vi "Buzzer.vi"   [LabVIEW 2022 SP3]
uses:
  <vilib>/DAQmx/write.llb/DAQmx Write (Digital Bool 1Line 1Point).vi
  <vilib>/DAQmx/create/channels.llb/DAQmx Create Channel (DO-Digital Output).vi
  <vilib>/DAQmx/miscellaneous.llb/DAQmx Fill In Error Info.vi
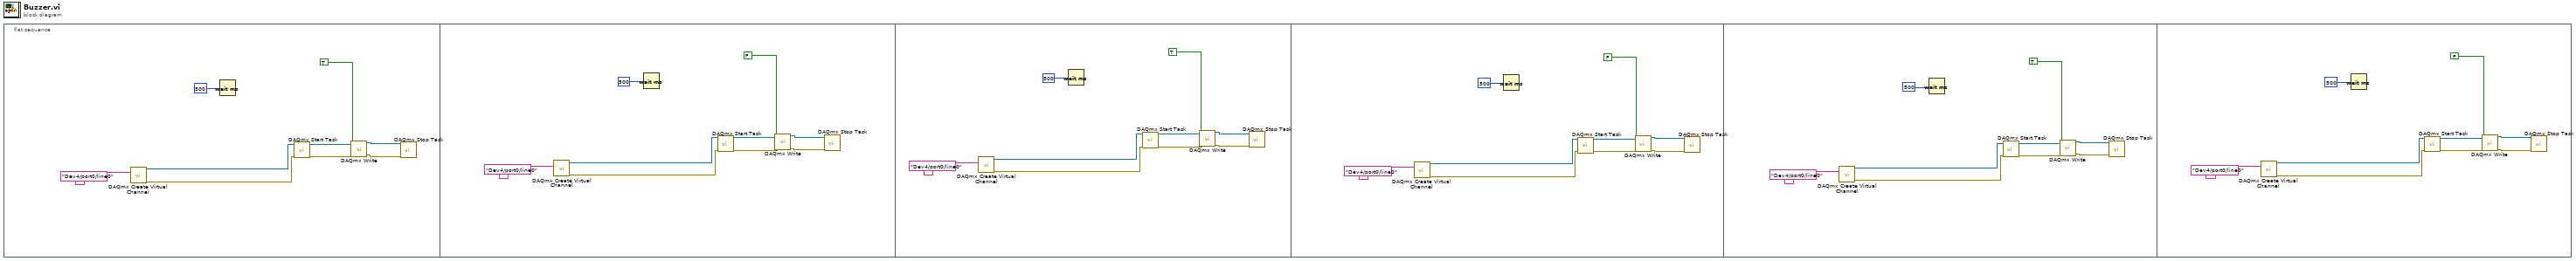
[diagram p0: block diagram]
diagram:
  n1 = flat-sequence {
    frame #0 {
      n2 = call-poly <vilib>:"DAQmx Create Virtual Channel.vi"("lines"=tag "Dev4/port0/line0" ("DAQmx Physical Channel")) -> ("task out"=w1:refnum<k21>, "error out"=w2:errorcluster)  [unwired: 13 in]
      n3 = Wait (ms)(milliseconds to wait=u32 500 ("millisecond timer value")) -> ()  [unwired: 1 out]
      n4 = call <vilib>:"DAQmx Start Task.vi"("task/channels in"=w1, "error in"=w2) -> ("task out"=w8:refnum<k21>, "error out"=w7:errorcluster)  [unwired: 12 in]
      n5 = call-poly <vilib>:"DAQmx Write.vi"("task/channels in"=w8, "data"=TRUE, "error in"=w7) -> ("task out"=w5:refnum<k21>, "error out"=w4:errorcluster)  [unwired: 10 in, 1 out]
      n6 = call <vilib>:"DAQmx Stop Task.vi"("task/channels in"=w5, "error in"=w4) -> ()  [unwired: 12 in, 2 out]
    }
    frame #1 {
      n7 = call-poly <vilib>:"DAQmx Create Virtual Channel.vi"("lines"=tag "Dev4/port0/line0" ("DAQmx Physical Channel")) -> ("task out"=w10:refnum<k21>, "error out"=w11:errorcluster)  [unwired: 13 in]
      n8 = Wait (ms)(milliseconds to wait=u32 500 ("millisecond timer value")) -> ()  [unwired: 1 out]
      n9 = call <vilib>:"DAQmx Start Task.vi"("task/channels in"=w10, "error in"=w11) -> ("task out"=w17:refnum<k21>, "error out"=w16:errorcluster)  [unwired: 12 in]
      n10 = call-poly <vilib>:"DAQmx Write.vi"("task/channels in"=w17, "data"=FALSE, "error in"=w16) -> ("task out"=w14:refnum<k21>, "error out"=w13:errorcluster)  [unwired: 10 in, 1 out]
      n11 = call <vilib>:"DAQmx Stop Task.vi"("task/channels in"=w14, "error in"=w13) -> ()  [unwired: 12 in, 2 out]
    }
    frame #2 {
      n12 = call-poly <vilib>:"DAQmx Create Virtual Channel.vi"("lines"=tag "Dev4/port0/line0" ("DAQmx Physical Channel")) -> ("task out"=w19:refnum<k21>, "error out"=w20:errorcluster)  [unwired: 13 in]
      n13 = Wait (ms)(milliseconds to wait=u32 500 ("millisecond timer value")) -> ()  [unwired: 1 out]
      n14 = call <vilib>:"DAQmx Start Task.vi"("task/channels in"=w19, "error in"=w20) -> ("task out"=w26:refnum<k21>, "error out"=w25:errorcluster)  [unwired: 12 in]
      n15 = call-poly <vilib>:"DAQmx Write.vi"("task/channels in"=w26, "data"=TRUE, "error in"=w25) -> ("task out"=w23:refnum<k21>, "error out"=w22:errorcluster)  [unwired: 10 in, 1 out]
      n16 = call <vilib>:"DAQmx Stop Task.vi"("task/channels in"=w23, "error in"=w22) -> ()  [unwired: 12 in, 2 out]
    }
    frame #3 {
      n17 = call-poly <vilib>:"DAQmx Create Virtual Channel.vi"("lines"=tag "Dev4/port0/line0" ("DAQmx Physical Channel")) -> ("task out"=w28:refnum<k21>, "error out"=w29:errorcluster)  [unwired: 13 in]
      n18 = Wait (ms)(milliseconds to wait=u32 500 ("millisecond timer value")) -> ()  [unwired: 1 out]
      n19 = call <vilib>:"DAQmx Start Task.vi"("task/channels in"=w28, "error in"=w29) -> ("task out"=w35:refnum<k21>, "error out"=w34:errorcluster)  [unwired: 12 in]
      n20 = call-poly <vilib>:"DAQmx Write.vi"("task/channels in"=w35, "data"=FALSE, "error in"=w34) -> ("task out"=w32:refnum<k21>, "error out"=w31:errorcluster)  [unwired: 10 in, 1 out]
      n21 = call <vilib>:"DAQmx Stop Task.vi"("task/channels in"=w32, "error in"=w31) -> ()  [unwired: 12 in, 2 out]
    }
    frame #4 {
      n22 = call-poly <vilib>:"DAQmx Create Virtual Channel.vi"("lines"=tag "Dev4/port0/line0" ("DAQmx Physical Channel")) -> ("task out"=w37:refnum<k21>, "error out"=w38:errorcluster)  [unwired: 13 in]
      n23 = Wait (ms)(milliseconds to wait=u32 500 ("millisecond timer value")) -> ()  [unwired: 1 out]
      n24 = call <vilib>:"DAQmx Start Task.vi"("task/channels in"=w37, "error in"=w38) -> ("task out"=w44:refnum<k21>, "error out"=w43:errorcluster)  [unwired: 12 in]
      n25 = call-poly <vilib>:"DAQmx Write.vi"("task/channels in"=w44, "data"=TRUE, "error in"=w43) -> ("task out"=w41:refnum<k21>, "error out"=w40:errorcluster)  [unwired: 10 in, 1 out]
      n26 = call <vilib>:"DAQmx Stop Task.vi"("task/channels in"=w41, "error in"=w40) -> ()  [unwired: 12 in, 2 out]
    }
    frame #5 {
      n27 = call-poly <vilib>:"DAQmx Create Virtual Channel.vi"("lines"=tag "Dev4/port0/line0" ("DAQmx Physical Channel")) -> ("task out"=w46:refnum<k21>, "error out"=w47:errorcluster)  [unwired: 13 in]
      n28 = Wait (ms)(milliseconds to wait=u32 500 ("millisecond timer value")) -> ()  [unwired: 1 out]
      n29 = call <vilib>:"DAQmx Start Task.vi"("task/channels in"=w46, "error in"=w47) -> ("task out"=w53:refnum<k21>, "error out"=w52:errorcluster)  [unwired: 12 in]
      n30 = call-poly <vilib>:"DAQmx Write.vi"("task/channels in"=w53, "data"=FALSE, "error in"=w52) -> ("task out"=w50:refnum<k21>, "error out"=w49:errorcluster)  [unwired: 10 in, 1 out]
      n31 = call <vilib>:"DAQmx Stop Task.vi"("task/channels in"=w50, "error in"=w49) -> ()  [unwired: 12 in, 2 out]
    }
  }
